vi "RegistredDataExample.vi"() -> ()   [LabVIEW 2009]
panel:
  in  "location":string="/TestData"
  in  "error in (no error)":errorcluster
  out "error out":errorcluster
  in  "compressionLevel":i32
  in  "elementDescription":string[](array[string])
  in  "initial data":dbl[](array[numeric])
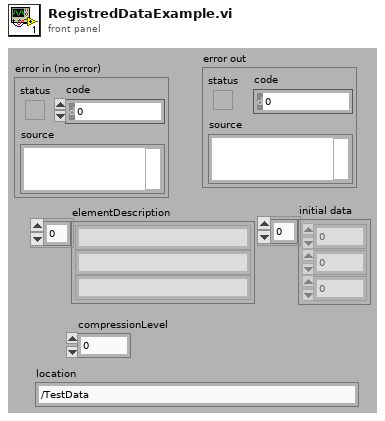
[diagram p1: front panel]
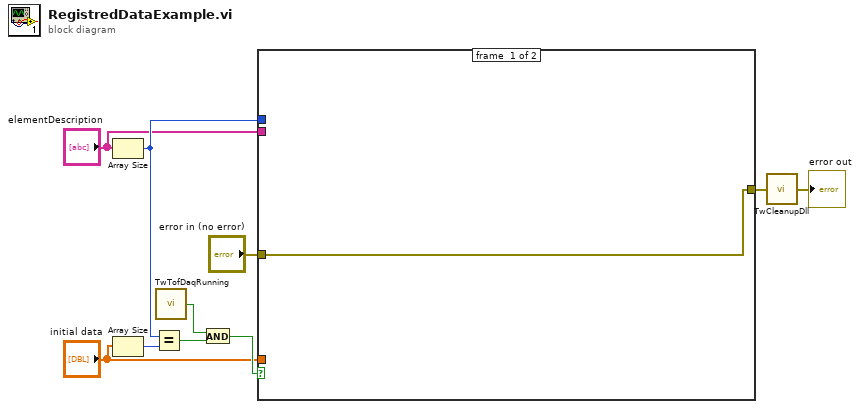
[diagram p0: block diagram]
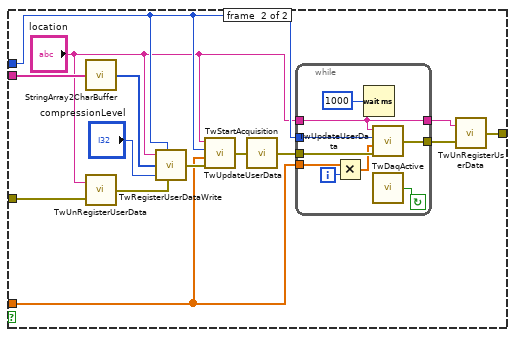
[diagram p2: hidden frame]
diagram:
  n1 = Array Size(array="elementDescription") -> (size(s)=w6:i32)
  n2 = Array Size(array="initial data") -> (size(s)=w7:i32)
  n3 = Equal?(x=w6, y=w7) -> (x = y?=w9:bool)
  n4 = call "TwTofDaqRunning.vi"() -> ("running?"=w10:bool)
  n5 = And(x=w10, y=w9) -> (x .and. y?=w8:bool)
  n6 = case shown="False" w8 {
    tunnel: w6 -> [_ w18]
    tunnel: "initial data" -> [_ w19]
    tunnel: "elementDescription" -> [_ w25]
    tunnel: [w11 w15] -> w3
    tunnel: "error in (no error)" -> [w11 w13]
    frame #0 {
    }
    frame #1 {
      n7 = call "StringArray2CharBuffer.vi"("elementDescription"=w25) -> ("Array"=w23:u8[])
      n8 = call "TwUnRegisterUserData.vi"("error in (no error)"=w13, "location"="location") -> ("error out"=w14:errorcluster)
      n9 = call "TwRegisterUserDataWrite.vi"("location"="location", "nbrElements"=w18, "elementDescription"=w23, "compressionLevel"="compressionLevel", "error in (no error)"=w14) -> ("error out"=w24:errorcluster)
      n10 = call "TwUpdateUserData.vi"("error in (no error)"=w24, "data"=w19, "nbrElements"=w18, "location"="location") -> ("error out"=w21:errorcluster)
      n11 = call "TwStartAcquisition.vi"("error in (no error)"=w21) -> ("error out"=w20:errorcluster)
      n12 = while {
        tunnel: w20 -> [w33]
        tunnel: w19 -> [w31]
        tunnel: w18 -> [w32]
        tunnel: "location" -> [w26]
        tunnel: [w27] -> w17
        tunnel: [w26] -> w16
        i -> [w30]
        stop <- w34 continue-if-true
        n13 = Multiply(x=w31, y=w30) -> (x*y=w29:dbl[])
        n14 = Wait (ms)(milliseconds to wait=u32 1000) -> ()  [unwired: 1 out]
        n15 = call "TwUpdateUserData.vi"("error in (no error)"=w33, "data"=w29, "nbrElements"=w32, "location"=w26) -> ("error out"=w27:errorcluster)
        n16 = call "TwDaqActive.vi"() -> ("DAQ active?"=w34:bool)
      }
      n17 = call "TwUnRegisterUserData.vi"("error in (no error)"=w17, "location"=w16) -> ("error out"=w15:errorcluster)
    }
  }
  n18 = call "TwCleanupDll.vi"("error in (no error)"=w3) -> ("error out"=→"error out":errorcluster)
